vi "channel operation tests.vi"() -> ()   [LabVIEW 2013, in "TEC tests.lvlib"]
uses:
  TEC tests.lvlib
  <vilib>/NI/Tag Bus Module Framework/channel/channel classification.ctl
  configuration/TEC configuration.lvclass
  configuration/TEC configuration.lvclass/TEC configuration.ctl
  configuration/Write channels.vi
  <vilib>/NI/Tag Bus Module Framework/channel/TBM channel.lvclass
  <vilib>/NI/Tag Bus Module Framework/root configuration/TBM configuration.lvclass
panel:
  out "channels match":bool
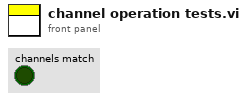
[diagram p1: front panel]
types:
  T1 = typedef "TBM channel.lvclass/channel classification.ctl" = enum16{"input data", "output data", "processing parameter", "processing result"}
  T2 = typedef "tag bus.lvlib/tag descriptor.lvclass/Data Type.ctl" = enum16{"Double", "Single", "I64", "I32", "I16", "I8", "U64", "U32", "U16", "U8", "Boolean", "String", "Array of Double", "Array of Single", "Array of I64", "Array of I32", "Array of I16", "Array of I8", "Array of U64", "Array of U32", "Array of U16", "Array of U8", "Array of Boolean", "Array of String"}
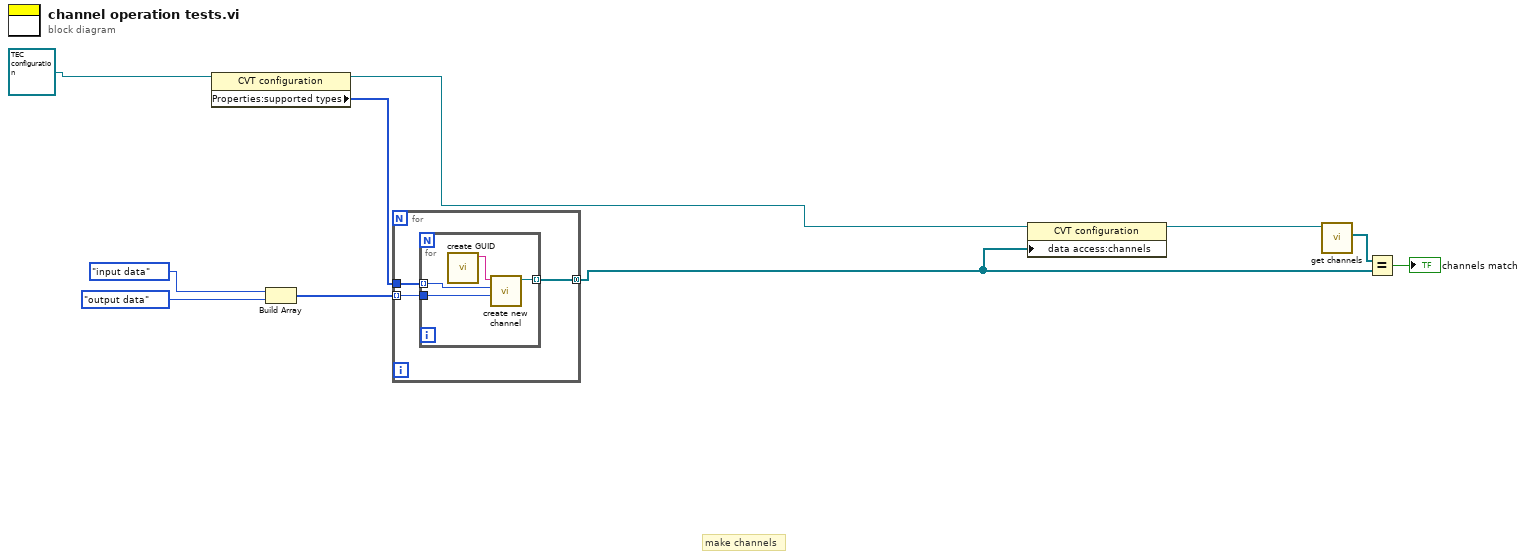
[diagram p0: block diagram]
diagram:
  # "make channels"
  n1 = property class="CVT configuration"(reference=refnum<class "TEC configuration.lvclass"> refnum ("tag bus configurable plugin module configuration")) -> (reference out=w7:refnum<class "TEC configuration.lvclass">, "Properties:supported types"=w6:T2[])  [unwired: 1 in, 1 out]
  n2 = Build Array(channel_classification."input data" ("channel classification"), channel_classification."output data" ("channel classification")) -> (w8:T1[])
  n3 = for {
    tunnel: w8 -> [w13] mode=indexing
    tunnel: [w11] -> w1 mode=concatenating
    tunnel: w6 -> [w12]
    n4 = for {
      tunnel: w13 -> [w16]
      tunnel: [w17] -> w11 mode=indexing
      tunnel: w12 -> [w15] mode=indexing
      n5 = call <vilib>:"create GUID.vi"() -> ("uuid"=w14:string)  [unwired: 11 in]
      n6 = call <vilib>:"create new channel.vi"("channel classification"=w16, "data type"=w15, "channel name"=w14) -> ("channel"=w17:refnum<class "TBM channel.lvclass">)  [unwired: 8 in]
    }
  }
  n7 = property class="CVT configuration"(reference=w7, "data access:channels"=w1) -> (reference out=w2:refnum<class "TEC configuration.lvclass">)  [unwired: 1 in, 1 out]
  n8 = call-dynamic "get channels.vi"("TEC configuration in"=w2) -> ("channels"=w5:refnum<class "TBM channel.lvclass">[])  [unwired: 9 in, 1 out]
  n9 = Equal?(x=w5, y=w1) -> (x = y?=→"channels match":bool)
